vi "z internal closure hello null.vi"(8 "error in (no error)":errorcluster, 11 "this_":cluster{"_context":u64, "_call":u64}) -> (0 "error out":errorcluster, 3 "this_ out":cluster{"_context":u64, "_call":u64})   [LabVIEW 2021, in "zenohc.lvlib"]
doc: "ZENOHC_API void z_internal_closure_hello_null(struct z_owned_closure_hello_t *this_);"
uses:
  zenohc.lvlib
  zenohc.dll
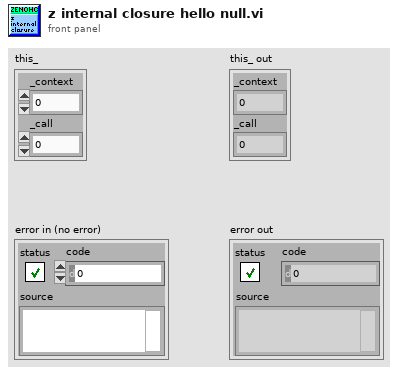
[diagram p1: front panel]
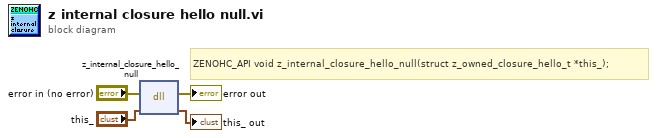
[diagram p0: block diagram]
diagram:
  # "ZENOHC_API void z_internal_closure_hello_null(struct z_owned_closure_hello_t *this_);"
  n1 = dll-call lib="D:/dev/zenoh_labview/zenohc/zenohc.*" fn="z_internal_closure_hello_null"(error in="error in (no error)", "this_"="this_") -> (error out=→"error out":errorcluster, "this_"=→"this_ out":cluster{"_context":u64, "_call":u64})  [unwired: 3 in, 1 out]
